vi "YKMW100 Get Error Log.vi"(0 "VISA session":refnum<visa-resource-name>="MW100", 9 "Timeout (25000)":u32=100, 11 "error in (no error)":errorcluster, 13 "Source (\"\")":string) -> (4 "dup VISA session":refnum<visa-resource-name>, 6 "Error History":string[](array[string]), 7 "Send Message (\"\")":string, 15 "error out":errorcluster)   [LabVIEW 2016]
doc: "This VI sends the message. Then it returns the response."
panel:
  out "Read Buffer":string
  in  "Number of Read Blocks (1-50)":i32
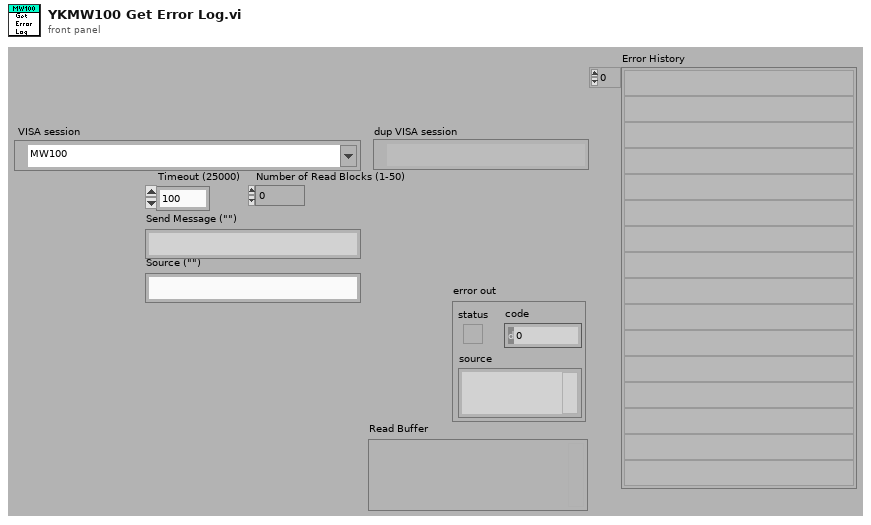
[diagram p1: front panel]
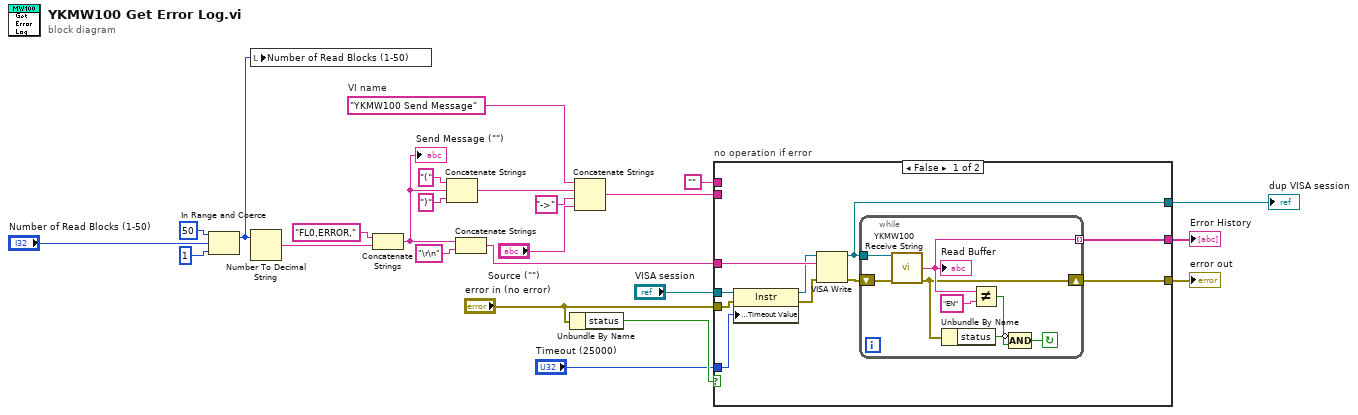
[diagram p0: block diagram]
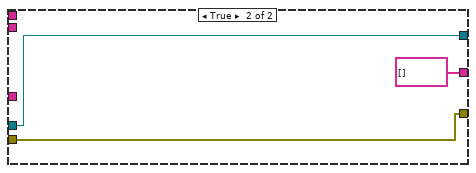
[diagram p2: hidden frame]
diagram:
  w14 = "YKMW100 Send Message"  # VI name
  n1 = In Range and Coerce(upper limit=50, x="Number of Read Blocks (1-50)", lower limit=1) -> (coerced(x)=w6:i32)  [unwired: 1 out]
  n2 = local write "Number of Read Blocks (1-50)"(w6) -> ()
  n3 = Number To Decimal String(number=w6) -> (decimal integer string=w5:string)  [unwired: 1 in]
  n4 = Concatenate Strings("FL0,ERROR,", w5) -> (w4:string)
  "Send Message (\"\")" <- w4
  n5 = Concatenate Strings("(", w4, ")") -> (w15:string)
  n6 = Concatenate Strings(w4, "\r\n") -> (w24:string)
  n7 = Unbundle By Name("error in (no error)") -> ("status"=w21:bool)
  n8 = Concatenate Strings(w14, w15, "->", "Source (\"\")") -> (w20:string)
  n9 = case "no operation if error" shown="False" w21 {
    tunnel: "VISA session" -> [w31 w45]
    tunnel: w24 -> [w34 _]
    tunnel: [w25 w45] -> w13
    tunnel: [w27 w44] -> w2
    tunnel: "error in (no error)" -> [w33 w44]
    tunnel: w20 -> [_ _]
    tunnel: "Timeout (25000)" -> [w29 _]
    tunnel: [w28 string[] []] -> w3
    tunnel: "" -> [_ _]
    frame False {
      n10 = property class="Instr"(reference=w31, error in=w33, "General Settings:Timeout Value"=w29) -> (reference out=w30:refnum<visa-resource-name>, error out=w32:errorcluster)
      n11 = VISA Write(VISA resource name=w30, write buffer=w34, error in (no error)=w32) -> (VISA resource name out=w25:refnum<visa-resource-name>, error out=w26:errorcluster)  [unwired: 1 out]
      n12 = while {
        tunnel: w25 -> [w42]
        tunnel: [w40] -> w28 mode=indexing
        shift-right: [w36] -> w27
        shift-left: w26 -> [w41]
        stop <- w37 continue-if-true
        n13 = call "YKMW100 Receive String.vi"("VISA session"=w42, "error in (no error)"=w41) -> ("Read Buffer"=w40:string, "error out"=w36:errorcluster)  [unwired: 11 in, 1 out]
        "Read Buffer" <- w40
        n14 = Unbundle By Name(w36) -> ("status"=w38:bool)
        n15 = Not Equal?(x=w40, y="EN" ("concatenated string")) -> (x != y?=w39:bool)
        n16 = Compound Arithmetic op=AND(invert w38, w39) -> (w37:bool)
      }
    }
    frame True {
    }
  }
  "error out" <- w2
  "dup VISA session" <- w13
  "Error History" <- w3
